vi "Delay Minutes.vi"(11 "Error In":errorcluster, 13 "minutes to wait":u32) -> (15 "Error Out":errorcluster)   [LabVIEW 2009]
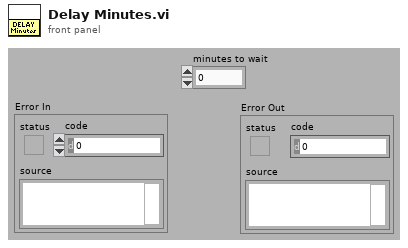
[diagram p1: front panel]
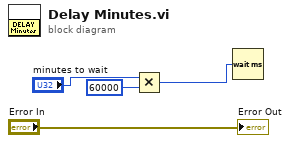
[diagram p0: block diagram]
diagram:
  n1 = Multiply(x="minutes to wait", y=u32 60000) -> (x*y=w1:u32)
  n2 = Wait (ms)(milliseconds to wait=w1) -> ()  [unwired: 1 out]
  "Error Out" <- "Error In"
